vi "Write CS++Factory.vi"(8 "Error In":errorcluster, 10 "CS++Factory":refnum<class "CS++Factory.lvclass">, 11 "CS++RTMainActor in":refnum<class "CS++RTMainActor.lvclass">) -> (0 "Error Out":errorcluster, 3 "CS++RTMainActor out":refnum<class "CS++RTMainActor.lvclass">)   [LabVIEW 2015, in "CS++RTMain.lvlib" / "CS++RTMainActor.lvclass"]
doc: "Write Factory to attribute."
uses:
  CS++RTMainActor.lvclass
  CSPP_Core/Classes/CS++BaseClasses/Factory/CS++Factory.lvclass
  CS++RTMainActor.lvclass/CS++RTMainActor.ctl
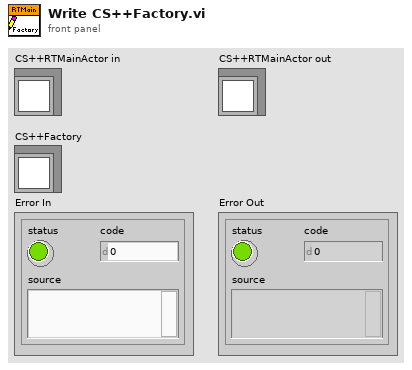
[diagram p1: front panel]
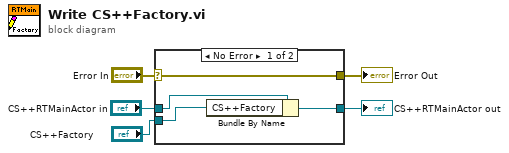
[diagram p0: block diagram]
diagram:
  n1 = case shown="No Error" "Error In" {
    selector: "Error In" -> [w9 w10]
    tunnel: [w9 w10] -> w4
    tunnel: [w7 w11] -> w2
    tunnel: "CS++RTMainActor in" -> [w8 w11]
    tunnel: "CS++Factory" -> [w6 _]
    frame No Error {
      n2 = Bundle By Name(cluster=w8, "CS++Factory"=w6) -> (w7:refnum<class "CS++RTMainActor.lvclass">)
    }
    frame Error {
    }
  }
  "Error Out" <- w4
  "CS++RTMainActor out" <- w2
